vi "Update Test Explanation.vi"(8 "error in (no error)":errorcluster, 10 "Test Explanation":T1, 11 "Test Event Storage in":refnum<class "Test Event Storage.lvclass">) -> (0 "error out":errorcluster, 3 "Test Event Storage out":refnum<class "Test Event Storage.lvclass">)   [LabVIEW 2013, in "Caraya.lvlib" / "Test Event Storage.lvclass"]
uses:
  Test Event Storage.lvclass
  Test Result/Test Verbose Explanation.ctl
  Test Event Storage.lvclass/Test Event Storage.ctl
  Test Result/Assert Event Data.ctl
  Test Result/Test Result.lvclass
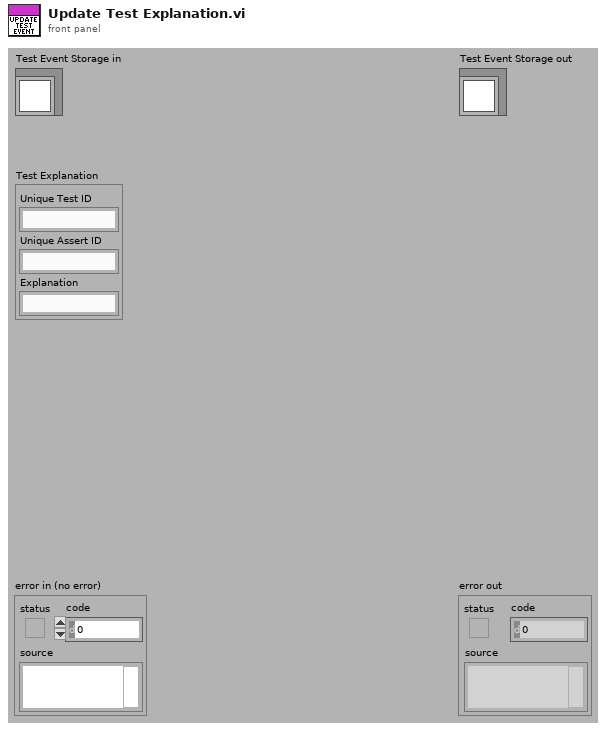
[diagram p1: front panel]
types:
  T1 = typedef "Caraya.lvlib/Test Result.lvclass/Test Verbose Explanation.ctl" = cluster{"Unique Test ID":string, "Unique Assert ID":string, "Explanation":string}
  T2 = typedef "Caraya.lvlib/Test Result.lvclass/Assert Event Data.ctl" = cluster{"Name":string, "Passed":bool, "Call Chain":string[], "Test Error":errorcluster, "Time Stamp":timestamp, "Unique Assert ID":string, "Test ID":string, "Execution time (s)":dbl, "Verbose Explanation":string}
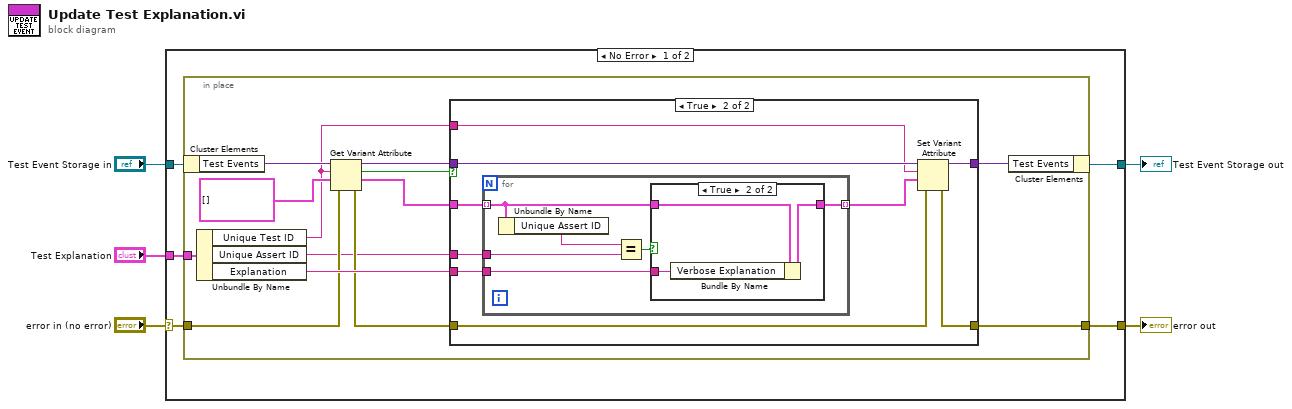
[diagram p0: block diagram]
diagram:
  n1 = case shown="No Error" "error in (no error)" {
    selector: "error in (no error)" -> [w6 w46]
    tunnel: [w10 w46] -> w4
    tunnel: [w9 w45] -> w2
    tunnel: "Test Event Storage in" -> [w7 w45]
    tunnel: "Test Explanation" -> [w8 _]
    frame No Error {
      n2 = in-place {
        in-place-border: w6 -> [w14]
        in-place-border: w8 -> [w20]
        in-place-border: [w22] -> w10
        n3 = in-place-cluster #1(w7) -> ("Test Events"=w19:variant)
        n4 = Unbundle By Name(w20) -> ("Unique Test ID"=w11:string, "Unique Assert ID"=w12:string, "Explanation"=w18:string)
        n5 = Get Variant Attribute(Variant=w19, name=w11, default value (empty Variant)=T2[] [], error in=w14) -> (duplicate Variant=w21:variant, found=w17:bool, value=w15:T2[], error out=w13:errorcluster)
        n6 = case shown="True" w17 {
          tunnel: [w25 w34] -> w23
          tunnel: [w24 w33] -> w22
          tunnel: w13 -> [w24 w32]
          tunnel: w21 -> [w25 w31]
          tunnel: w11 -> [_ w30]
          tunnel: w15 -> [_ w29]
          tunnel: w18 -> [_ w28]
          tunnel: w12 -> [_ w26]
          frame False {
          }
          frame True {
            n7 = for {
              tunnel: w29 -> [w38] mode=indexing
              tunnel: w28 -> [w40]
              tunnel: [w39] -> w27 mode=indexing
              tunnel: w26 -> [w36]
              n8 = Unbundle By Name(w38) -> ("Unique Assert ID"=w37:string)
              n9 = Equal?(x=w37, y=w36) -> (x = y?=w35:bool)
              n10 = case shown="True" w35 {
                tunnel: w40 -> [_ w44]
                tunnel: [w41 w43] -> w39
                tunnel: w38 -> [w41 w42]
                frame False {
                }
                frame True {
                  n11 = Bundle By Name(cluster=w42, "Verbose Explanation"=w44) -> (w43:T2)
                }
              }
            }
            n12 = Set Variant Attribute(Variant=w31, name=w30, value=w27, error in=w32) -> (Variant out=w34:variant, error out=w33:errorcluster)  [unwired: 1 out]
          }
        }
        n13 = in-place-cluster #1("Test Events"=w23) -> (w9:refnum<class "Test Event Storage.lvclass">)
      }
    }
    frame Error {
    }
  }
  "error out" <- w4
  "Test Event Storage out" <- w2
